vi "postprocess.vi"(8 "error in (no error)":errorcluster, 10 "segmented image file path in":path, 11 "SegmenterDL100224ThreeD in":refnum<class "SegmenterDL100224ThreeD.lvclass">) -> (0 "error out":errorcluster, 1 "centroids file path":path, 2 "segmented image path out":path, 3 "SegmenterDL100224ThreeD out":refnum<class "SegmenterDL100224ThreeD.lvclass">)   [LabVIEW 2010, in "SegmenterDL100224ThreeD.lvclass"]
uses:
  SegmenterDL100224ThreeD.lvclass
panel:
  out "console input":string
  out "console output":string
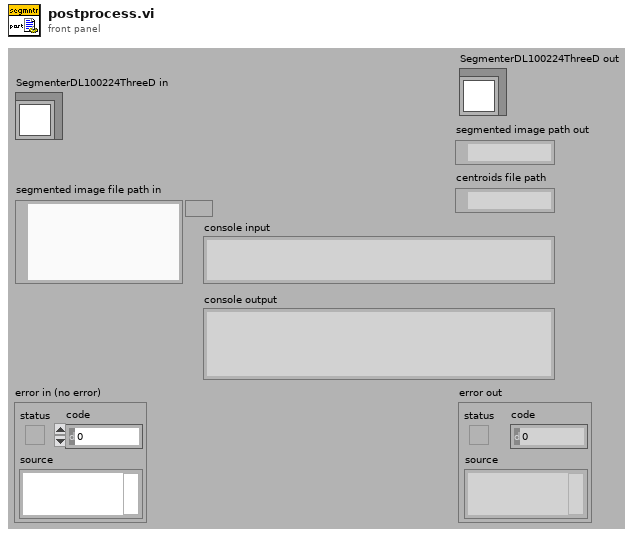
[diagram p1: front panel]
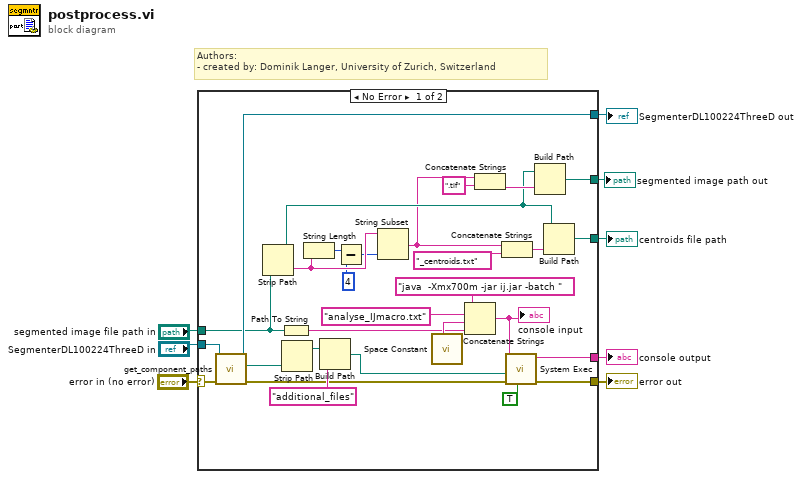
[diagram p0: block diagram]
diagram:
  # "Authors: \n- created by: Dominik Langer, University of Zurich, Switzerland"
  n1 = case shown="No Error" "error in (no error)" {
    selector: "error in (no error)" -> [w15 w39]
    tunnel: [w27 w39] -> w3
    tunnel: [w28 w38] -> w4
    tunnel: "SegmenterDL100224ThreeD in" -> [w29 w38]
    tunnel: "segmented image file path in" -> [w14 _]
    tunnel: [w23 _] -> w2
    tunnel: [w16 _] -> w5
    tunnel: [w10 _] -> w1
    frame No Error {
      n2 = call-dynamic "get_component_paths.vi"("error in (no error)"=w15, "GenericComponent in"=w29) -> ("error out"=w33:errorcluster, "specific component directory"=w32:path, "GenericComponent out"=w28:refnum<class "SegmenterDL100224ThreeD.lvclass">)  [unwired: 4 in, 3 out]
      n3 = Strip Path(path=w14) -> (stripped path=w11:path, name=w22:string)
      n4 = Path To String(path=w14) -> (string=w30:string)
      n5 = Strip Path(path=w32) -> (stripped path=w36:path)  [unwired: 1 out]
      n6 = String Length(string=w22) -> (length=w21:i32)
      n7 = Build Path(base path=w36, name or relative path="additional_files") -> (appended path=w24:path)
      n8 = Subtract(x=w21, y=4) -> (x-y=w19:i32)
      n9 = String Subset(string=w22, length (rest)=w19) -> (substring=w9:string)  [unwired: 1 in]
      n10 = call <vilib>:"Space Constant.vi"() -> ("String"=w31:string)
      n11 = Concatenate Strings("java  -Xmx700m -jar ij.jar -batch ", "analyse_IJmacro.txt" ("name or relative path"), w31, w30) -> (w34:string)
      "console input" <- w34
      n12 = Concatenate Strings(w9, ".tif" ("string")) -> (w12:string)
      n13 = Concatenate Strings(w9, "_centroids.txt" ("string")) -> (w18:string)
      n14 = call <vilib>:"System Exec.vi"("run minimized? (F)"=TRUE, "error in (no error)"=w33, "working directory"=w24, "command line"=w34) -> ("error out"=w27:errorcluster, "standard output"=w23:string)  [unwired: 4 in, 2 out]
      n15 = Build Path(base path=w11, name or relative path=w12) -> (appended path=w10:path)
      n16 = Build Path(base path=w11, name or relative path=w18) -> (appended path=w16:path)
    }
    frame Error {
    }
  }
  "error out" <- w3
  "SegmenterDL100224ThreeD out" <- w4
  "centroids file path" <- w5
  "console output" <- w2
  "segmented image path out" <- w1
